vi "getMeterProps.vi"(9 "array of frequencies":dbl[](array[numeric]), 11 "Detected frequency":dbl=320.0 format="%#_13g") -> (0 "BGColor":u32, 2 "Detected string":T1, 3 "Closest frequency":dbl, 4 "ScaleMax":i32, 6 "ScaleMin":i32)   [LabVIEW 2019]
uses:
  Strings.ctl
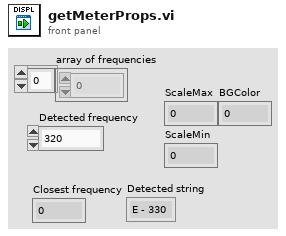
[diagram p1: front panel]
types:
  T1 = typedef "Strings.ctl" = enum16{"E - 330", "H - 247", "G - 196", "D - 147", "A - 110", "E - 82"}
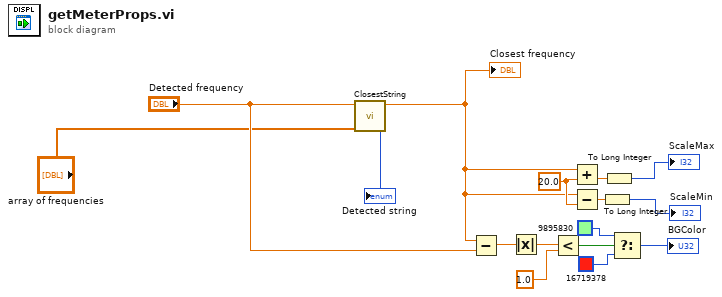
[diagram p0: block diagram]
diagram:
  w15 = 20.0 ("y")
  n1 = call "ClosestString.vi"("array of frequencies"="array of frequencies", "Detected frequency"="Detected frequency") -> ("Closest string"=→"Detected string":T1, "Closest frequecny"=w6:dbl)  [unwired: 7 in, 1 out]
  "Closest frequency" <- w6
  n2 = Subtract(x=w6, y="Detected frequency") -> (x-y=w9:dbl)
  n3 = Absolute Value(x=w9) -> (abs(x)=w8:dbl)
  n4 = Less?(x=w8, y=1.0) -> (x < y?=w12:bool)
  n5 = Add(x=w6, y=w15) -> (x+y=w14:dbl)
  n6 = Subtract(x=w6, y=w15) -> (x-y=w13:dbl)
  n7 = To Long Integer(number=w13) -> (32bit integer=→"ScaleMin":i32)
  n8 = To Long Integer(number=w14) -> (32bit integer=→"ScaleMax":i32)
  n9 = Select(t=u32 9895830, s=w12, f=u32 16719378) -> (s? t:f=→"BGColor":u32)
